vi "KeDSO Setup Virtual Channels.vi"(6 "trigger config":T1, 7 "ranges override [Vpk] (default: empty)":dbl[](array[numeric]), 8 "error in":errorcluster, 9 "samples count (1000)":i64=1000, 10 "fs [Hz] (1M)":dbl=1000000.0, 11 "keysight dso":T3 {"bw limit [Hz]" format="%#_6p"; "channels"."Offset [V]" min=0.0 format="%#_6p"; "channels"."Range [Vpk]" min=0.0 format="%#_6p"; "channels"."Channel" min=1}) -> (0 "error out":errorcluster, 3 "keysight dso out":T3 {"bw limit [Hz]" format="%#_6p"; "channels"."Offset [V]" min=0.0 format="%#_6p"; "channels"."Range [Vpk]" min=0.0 format="%#_6p"; "channels"."Channel" min=1})   [LabVIEW 2020]
doc: "Sets Keysight DSO virtual digitizer for sampling. Call at least once before acquisition."
uses:
  KeDSO session.ctl
  KeDSO Virtual Channel.ctl
  KeDSO Trigger Setup.ctl
  KeDSO Trigger Source.ctl
  <vilib>/Utility/error.llb/Error Cluster From Error Code.vi
  Public/Configure/Trigger/Configure Trigger (Edge).vi
  Public/Configure/Trigger/Configure Trigger (Timeout).vi
  <vilib>/ErrorRing/Error Ring.xnode
  Agilent 90000 Series.lvlib
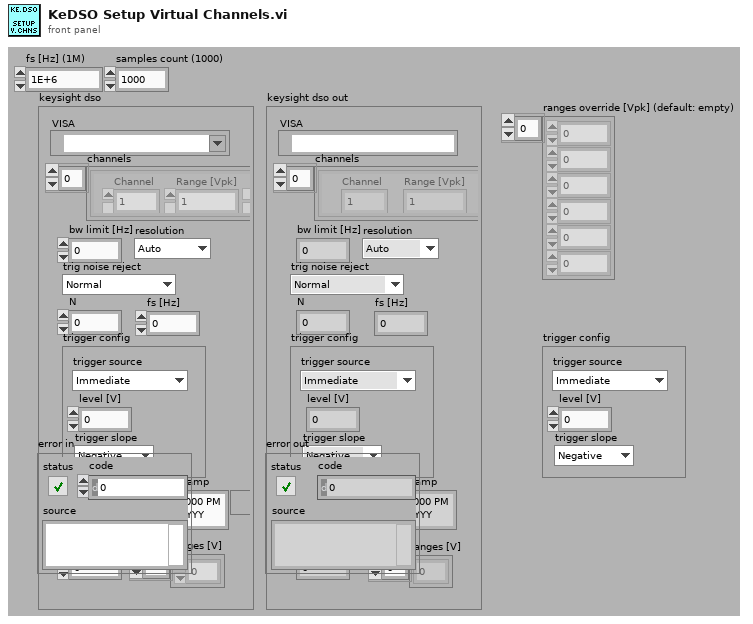
[diagram p1: front panel]
types:
  T1 = typedef "KeDSO Trigger Setup.ctl" = cluster{"trigger source":T2, "level [V]":dbl, "trigger slope":enum16{"Negative", "Positive", "Either"}}
  T2 = typedef "KeDSO Trigger Source.ctl" = enum16{"Immediate", "Level", "AUX"}
  T3 = typedef "KeDSO session.ctl" = cluster{"VISA":refnum<visa-resource-name>, "channels":T4[], "bw limit [Hz]":dbl, "resolution":enum16{"Auto", "Bits 9", "Bits 10", "Bits 11", "Bits 12"}, "trig noise reject":enum16{"Normal", "High Sensitivity"}, "N":i64, "trigger config":T1, "fs [Hz]":dbl, "timeout stop":timestamp, "waiting for opc":bool, "fetch offset [smpl]":i64, "abs timestamp":timestamp, "ranges [V]":dbl[]}
  T4 = typedef "KeDSO Virtual Channel.ctl" = cluster{"Channel":i32, "Range [Vpk]":dbl, "btn clr":bool, "btn up":bool, "btn down":bool, "Offset [V]":dbl, "Coupling":enum16{"DC", "DC50", "AC", "LFR1"}, "bw limit enab":bool}
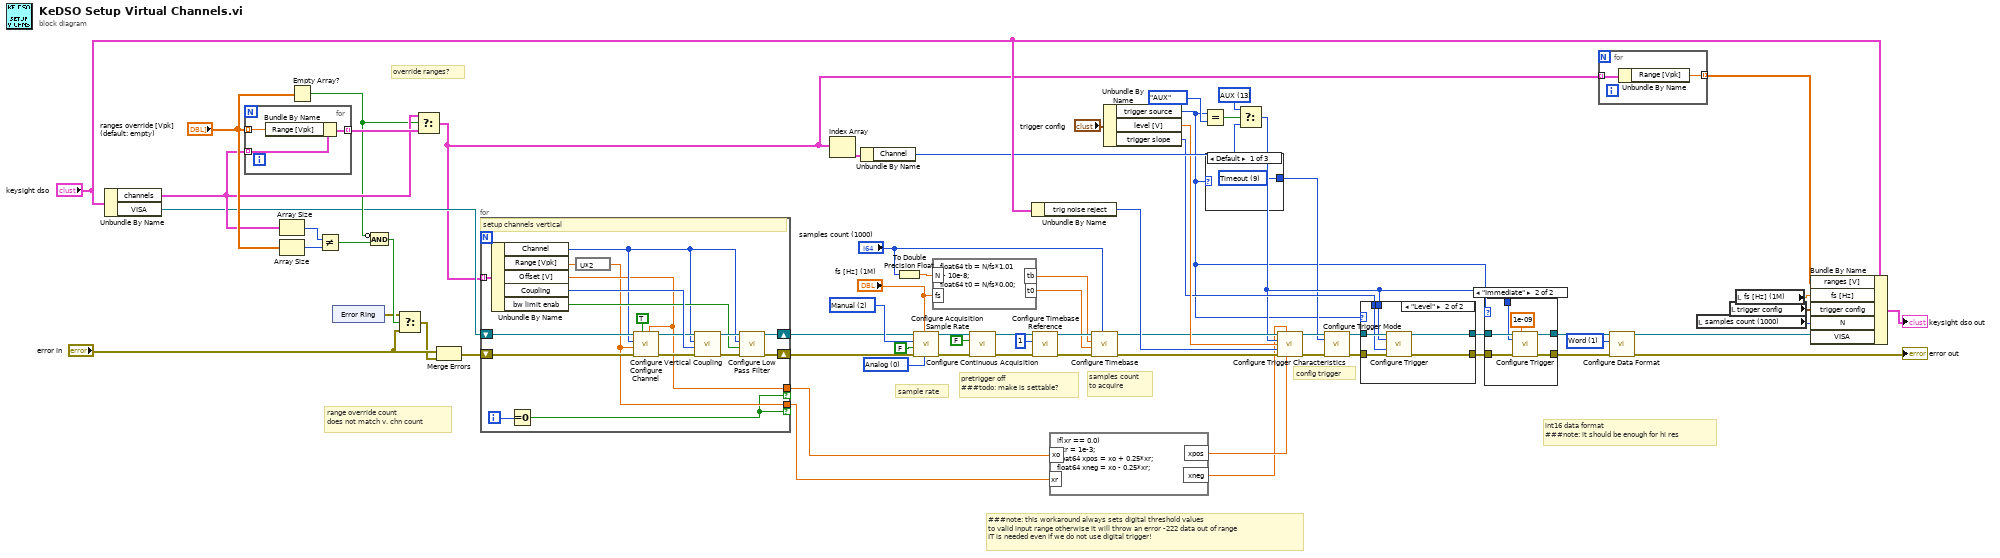
[diagram p0: block diagram]
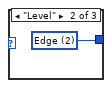
[diagram p4: hidden frame]
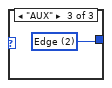
[diagram p5: hidden frame]
diagram:
  w29 = 1 items=["Byte", "Word"] ("Data Format (0: Byte)")
  w38 = 13 items=["Channel1"=1, "Channel2"=2, "Channel3"=3, "Channel4"=4, "AUX"=13] ("Trigger Source (1: Channel1)")
  w64 = u16 0 items=["Analog", "Digital"] ("Setting Type (0: Analog)")
  w66 = 2 items=["Auto", "Max", "Manual"] ("Sample Rate Method (0: Auto)")
  # "###note: this workaround always sets digital threshold values\nto valid input range otherwise it will throw an error -222 data out of range\nIT is needed even if we do not use digital trigger!"
  # "int16 data format\n###note: it should be enough for hi res"
  # "config trigger"
  # "samples count\nto acquire"
  # "pretrigger off\n###todo: make is settable?"
  # "sample rate"
  # "range override count\ndoes not match v. chn count"
  # "override ranges?"
  n1 = Unbundle By Name("keysight dso") -> ("channels"=w55:T4[], "VISA"=w28:refnum<visa-resource-name>)
  n2 = for {
    tunnel: w55 -> [w70] mode=indexing
    tunnel: "ranges override [Vpk] (default: empty)" -> [w69] mode=indexing
    tunnel: [w68] -> w56 mode=indexing
    n3 = Bundle By Name(cluster=w70, "Range [Vpk]"=w69) -> (w68:T4)
  }
  n4 = Array Size(array=w55) -> (size(s)=w58:i32)
  n5 = Array Size(array="ranges override [Vpk] (default: empty)") -> (size(s)=w59:i32)
  n6 = Empty Array?(array="ranges override [Vpk] (default: empty)") -> (empty?=w53:bool)
  n7 = Not Equal?(x=w58, y=w59) -> (x != y?=w54:bool)
  n8 = xnode "Error Ring"() -> ("error out"=w51:errorcluster)
  n9 = Compound Arithmetic op=AND(invert w53, w54) -> (w52:bool)
  n10 = Select(t=w51, s=w52, f="error in") -> (s? t:f=w49:errorcluster)
  n11 = Select(t=w55, s=w53, f=w56) -> (s? t:f=w24:T4[])
  n12 = Merge Errors("error in", w49) -> (w48:errorcluster)
  n13 = for {
    shift-right: [w78] -> w27
    shift-left: w28 -> [w87]
    shift-right: [w79] -> w47
    shift-left: w48 -> [w88]
    tunnel: w24 -> [w85] mode=indexing
    tunnel: [w74] -> w4 if=w71
    tunnel: [w72] -> w3 if=w71
    i -> [w73]
    # "setup channels vertical"
    n14 = Unbundle By Name(w85) -> ("Channel"=w75:i32, "Range [Vpk]"=w84:dbl, "Offset [V]"=w74:dbl, "Coupling"=w83:enum16{"DC", "DC50", "AC", "LFR1"}, "bw limit enab"=w80:bool)
    n15 = Equal To 0?(x=w73) -> (x = 0?=w71:bool)
    n16 = expression code="U*2"(w84) -> (w72:dbl)
    n17 = call "Configure Channel.vi"("Vertical Offset (0.0 V)"=w74, "Enable Channel (T: Enable)"=TRUE, "error in (no error)"=w88, "Vertical Range (2.0 V)"=w72, "Channel (1: Channel 1)"=w75, "VISA resource name"=w87) -> ("error out"=w77:errorcluster, "VISA resource name out"=w76:refnum<visa-resource-name>)  [unwired: 4 in]
    n18 = call "Configure Vertical Coupling.vi"("error in (no error)"=w77, "Vertical Coupling (0: DC)"=w83, "Channel (1: Channel 1)"=w75, "VISA resource name"=w76) -> ("error out"=w82:errorcluster, "VISA resource name out"=w81:refnum<visa-resource-name>)  [unwired: 6 in]
    n19 = call "Configure Low Pass Filter.vi"("error in (no error)"=w82, "Enable Limit Bandwidth (F: Disable)"=w80, "Channel (1: Channel 1)"=w75, "VISA resource name"=w81) -> ("error out"=w79:errorcluster, "VISA resource name out"=w78:refnum<visa-resource-name>)  [unwired: 6 in]
  }
  n20 = Index Array(array=w24) -> (element=w60:T4)  [unwired: 1 in]
  n21 = Unbundle By Name(w60) -> ("Channel"=w36:i32)
  n22 = To Double Precision Float(number="samples count (1000)") -> (double precision float=w16:dbl)
  n23 = call "Configure Acquisition Sample Rate.vi"("Setting Type (0: Analog)"=w64, "Sample Rate (0)"="fs [Hz] (1M)", "error in (no error)"=w47, "Automatic Sampling Rate (T: Enable)"=FALSE, "Sample Rate Method (0: Auto)"=w66, "VISA resource name"=w27) -> ("error out"=w63:errorcluster, "VISA resource name out"=w62:refnum<visa-resource-name>)  [unwired: 4 in]
  n24 = formula code="float64 tb = N/fs*1.01 + 10e-8;\nfloat64 t0 = N/fs*0.00;"("N"=w16, "fs"="fs [Hz] (1M)") -> ("tb"=w15:dbl, "t0"=w9:dbl)
  n25 = call "Configure Continuous Acquisition.vi"("error in (no error)"=w63, "Enable Continuous Acquisition Mode (T:Enable)"=FALSE, "VISA resource name"=w62) -> ("error out"=w46:errorcluster, "VISA resource name out"=w44:refnum<visa-resource-name>)  [unwired: 7 in]
  n26 = Unbundle By Name("keysight dso") -> ("trig noise reject"=w42:enum16{"Normal", "High Sensitivity"})
  n27 = call "Configure Timebase Reference.vi"("error in (no error)"=w46, "Reference Position Percent (50)"=1, "VISA resource name"=w44) -> ("error out"=w22:errorcluster, "VISA resource name out"=w19:refnum<visa-resource-name>)  [unwired: 7 in]
  n28 = formula code="if(xr == 0.0)\n  xr = 1e-3;\nfloat64 xpos = xo + 0.25*xr;\nfloat64 xneg = xo - 0.25*xr;"("xo"=w4, "xr"=w3) -> ("xpos"=w2:dbl, "xneg"=w1:dbl)
  n29 = call "Configure Timebase.vi"("Record Length (1000)"="samples count (1000)", "error in (no error)"=w22, "Position (0.0 s)"=w9, "Timebase (0.005 s)"=w15, "VISA resource name"=w19) -> ("error out"=w21:errorcluster, "VISA resource name out"=w20:refnum<visa-resource-name>)  [unwired: 5 in]
  n30 = Unbundle By Name("trigger config") -> ("trigger source"=w7:T2, "level [V]"=w35:dbl, "trigger slope"=w30:enum16{"Negative", "Positive", "Either"})
  n31 = Equal?(x=w7, y=KeDSO_Trigger_Source."AUX") -> (x = y?=w37:bool)
  n32 = case shown="Default" w7 {
    tunnel: [w89 w90 w91] -> w8
    frame Default {
      w89 = 9 items=["Communication", "Delay", "Edge ", "Glitch", "Pattern", "Pulse Width ", "Runt", "Setup and Hold Time", "State", "Timeout", "Transition", "TV", "Window", "Advanced", "Serial Bus 1", "Serial Bus 2", "Serial Bus 3", "Serial Bus 4"] ("Trigger Mode (2: Edge)")
    }
    frame "Level" {
      w90 = 2 items=["Communication", "Delay", "Edge ", "Glitch", "Pattern", "Pulse Width ", "Runt", "Setup and Hold Time", "State", "Timeout", "Transition", "TV", "Window", "Advanced", "Serial Bus 1", "Serial Bus 2", "Serial Bus 3", "Serial Bus 4"] ("Trigger Mode (2: Edge)")
    }
    frame "AUX" {
      w91 = 2 items=["Communication", "Delay", "Edge ", "Glitch", "Pattern", "Pulse Width ", "Runt", "Setup and Hold Time", "State", "Timeout", "Transition", "TV", "Window", "Advanced", "Serial Bus 1", "Serial Bus 2", "Serial Bus 3", "Serial Bus 4"] ("Trigger Mode (2: Edge)")
    }
  }
  n33 = Select(t=w38, s=w37, f=w36) -> (s? t:f=w10:i32)
  n34 = call "Configure Trigger Characteristics.vi"("VISA resource name"=w20, "Low Threshold Voltage (-0.2 V)"=w1, "Trigger Source (1: Channel1)"=w10, "Trigger Level (0.0 V)"=w35, "Noise Reject Type (0: Normal)"=w42, "error in (no error)"=w21, "High Threshold Voltage (0 V)"=w2) -> ("VISA resource name out"=w33:refnum<visa-resource-name>, "error out"=w34:errorcluster)  [unwired: 7 in]
  n35 = call "Configure Trigger Mode.vi"("VISA resource name"=w33, "Trigger Mode (2: Edge)"=w8, "error in (no error)"=w34) -> ("VISA resource name out"=w31:refnum<visa-resource-name>, "error out"=w32:errorcluster)  [unwired: 11 in]
  n36 = case shown="\"Level\"" w7 {
    tunnel: w32 -> [w92 w99]
    tunnel: w31 -> [w93 w98]
    tunnel: w30 -> [_ w97]
    tunnel: [w92 w95] -> w14
    tunnel: [w93 w94] -> w11
    tunnel: w10 -> [_ w96]
    frame Default {
    }
    frame "Level" {
      n37 = call-poly "Configure Trigger.vi"("VISA resource name"=w98, "Trigger Source (1: Channel1)"=w96, "Edge Trigger Slope (0: Negative)"=w97, "error in (no error)"=w99) -> ("VISA resource name out"=w94:refnum<visa-resource-name>, "error out"=w95:errorcluster)  [unwired: 10 in]
    }
  }
  n38 = case shown="\"Immediate\"" w7 {
    tunnel: w14 -> [w100 w107]
    tunnel: [w100 w106] -> w13
    tunnel: [w101 w105] -> w12
    tunnel: w11 -> [w101 w104]
    tunnel: w10 -> [_ w103]
    frame Default {
    }
    frame "Immediate" {
      n39 = call-poly "Configure Trigger.vi"("VISA resource name"=w104, "Time (1E-9 s)"=1e-09 ("Delay Time (3E-8 s)"), "Trigger Source (1: Channel1)"=w103, "error in (no error)"=w107) -> ("VISA resource name out"=w105:refnum<visa-resource-name>, "error out"=w106:errorcluster)  [unwired: 10 in]
    }
  }
  n40 = for {
    tunnel: w24 -> [w109] mode=indexing
    tunnel: [w108] -> w23 mode=indexing
    n41 = Unbundle By Name(w109) -> ("Range [Vpk]"=w108:dbl)
  }
  n42 = call "Configure Data Format.vi"("error in (no error)"=w13, "Data Format (0: Byte)"=w29, "VISA resource name"=w12) -> ("error out"=→"error out":errorcluster, "VISA resource name out"=w5:refnum<visa-resource-name>)  [unwired: 7 in]
  n43 = local read "samples count (1000)"() -> (w41:i64)
  n44 = local read "trigger config"() -> (w26:T1)
  n45 = local read "fs [Hz] (1M)"() -> (w25:dbl)
  n46 = Bundle By Name(cluster="keysight dso", "ranges [V]"=w23, "fs [Hz]"=w25, "trigger config"=w26, "N"=w41, "VISA"=w5) -> (→"keysight dso out":T3)
